vi "Write device_handle.vi"(8 "error in (no error)":errorcluster, 10 "device_handle":i32, 11 "Dali_usb_tridonics in":refnum<class "Dali_usb_tridonics.lvclass">) -> (0 "error out":errorcluster, 3 "Dali_usb_tridonics out":refnum<class "Dali_usb_tridonics.lvclass">)   [LabVIEW 2014, in "Driver_interaction.lvlib" / "Dali_usb_tridonics.lvclass"]
uses:
  Dali_usb_tridonics.lvclass
  Dali_usb_tridonics.lvclass/Dali_usb_tridonics.ctl
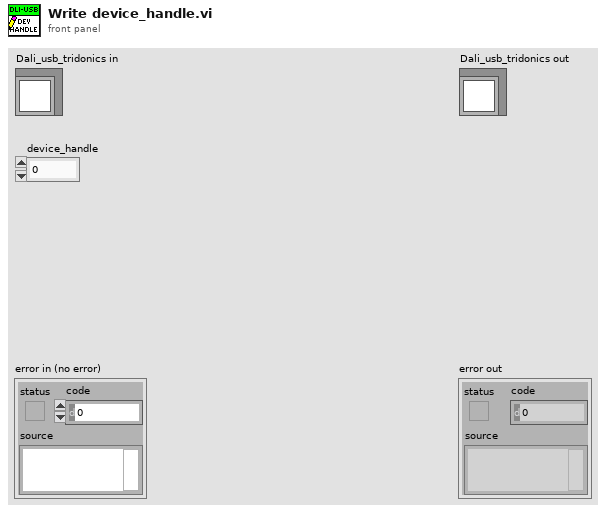
[diagram p1: front panel]
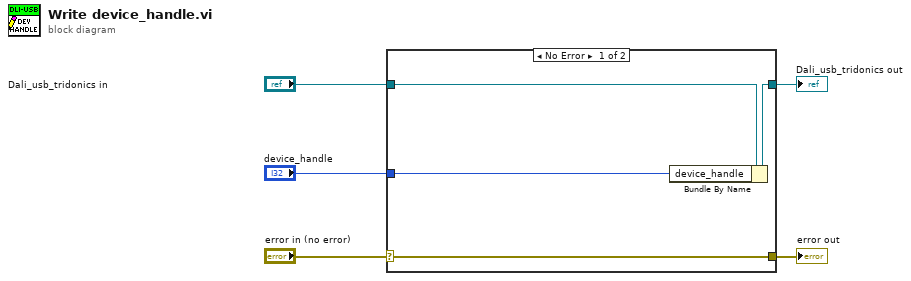
[diagram p0: block diagram]
diagram:
  n1 = case shown="No Error" "error in (no error)" {
    selector: "error in (no error)" -> [w9 w10]
    tunnel: [w9 w10] -> w4
    tunnel: [w7 w11] -> w2
    tunnel: "Dali_usb_tridonics in" -> [w8 w11]
    tunnel: "device_handle" -> [w6 _]
    frame No Error {
      n2 = Bundle By Name(cluster=w8, "device_handle"=w6) -> (w7:refnum<class "Dali_usb_tridonics.lvclass">)
    }
    frame Error {
    }
  }
  "error out" <- w4
  "Dali_usb_tridonics out" <- w2
